vi "Table Info.vi"(8 "error in (no error)":errorcluster, 10 "table":string, 11 "SQLite3LV Cursor in":refnum<class "cursor.lvclass">) -> (0 "error out":errorcluster, 2 "table info.":T1[](array[typedef]), 3 "SQLite3LV Cursor out":refnum<class "cursor.lvclass">)   [LabVIEW 2014, in "SQLite3LV.lvlib" / "cursor.lvclass"]
doc: "A utility function that returns information about the specified table."
uses:
  cursor.lvclass
  SQLite3 Class/struct_table_info.ctl
  property binding/column I32.vi
  property binding/column Text.vi
  SQLite3LV.lvlib
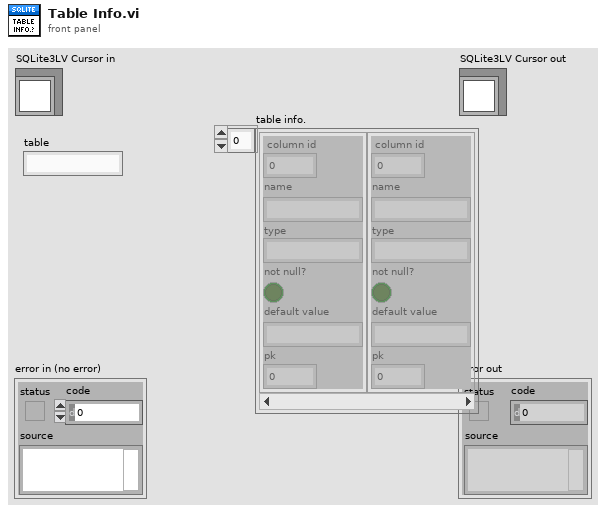
[diagram p1: front panel]
types:
  T1 = typedef "SQLite3LV.lvlib/struct_table_info.ctl" = cluster{" column id":i32, "name":string, "type":string, "not null?":bool, "default value":string, "pk":i32}
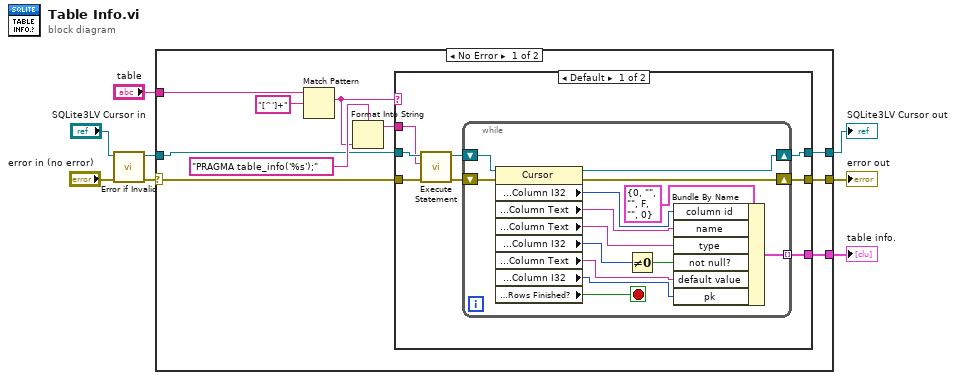
[diagram p0: block diagram]
diagram:
  n1 = call "Error if Invalid.vi"("error in (no error)"="error in (no error)", "SQLite3LV Cursor in"="SQLite3LV Cursor in") -> ("error out"=w1:errorcluster, "SQLite3LV Cursor out"=w2:refnum<class "cursor.lvclass">)  [unwired: 8 in]
  n2 = case shown="No Error" w1 {
    selector: w1 -> [w12 w44]
    tunnel: [w11 w44] -> w8
    tunnel: [w10 w43] -> w7
    tunnel: w2 -> [w13 w43]
    tunnel: "table" -> [w16 _]
    tunnel: [w9 _] -> w5
    frame No Error {
      n3 = Match Pattern(string=w16, regular expression="[^']+") -> (match substring=w15:string)  [unwired: 1 in, 3 out]
      n4 = Format Into String(format string="PRAGMA table_info('%s');", w15) -> (resulting string=w14:string)  [unwired: 2 in, 1 out]
      n5 = case shown="Default" w15 {
        tunnel: w14 -> [w25 _]
        tunnel: w13 -> [w26 w41]
        tunnel: w12 -> [w24 w42]
        tunnel: [w20 w42] -> w11
        tunnel: [w21 w41] -> w10
        tunnel: [w19 _] -> w9
        frame Default {
          n6 = call "Execute Statement.vi"("error in (no error)"=w24, "SQL statement"=w25, "SQLite3LV Cursor in"=w26) -> ("error out"=w22:errorcluster, "SQLite3LV Cursor out"=w23:refnum<class "cursor.lvclass">)  [unwired: 7 in]
          n7 = while {
            tunnel: [w32] -> w19 mode=indexing
            shift-right: [w29] -> w21
            shift-left: w23 -> [w40]
            shift-right: [w27] -> w20
            shift-left: w22 -> [w28]
            stop <- w31 stop-if-true
            n8 = property class="Cursor"(reference=w40, error in=w28) -> (reference out=w29:refnum<class "cursor.lvclass">, error out=w27:errorcluster, "property binding:Column I32"=w39:i32, "property binding:Column Text"=w35:string, "property binding:Column Text"=w36:string, "property binding:Column I32"=w38:i32, "property binding:Column Text"=w34:string, "property binding:Column I32"=w33:i32, "property binding:Rows Finished?"=w31:bool)
            n9 = Not Equal To 0?(x=w38) -> (x != 0?=w37:bool)
            n10 = Bundle By Name(cluster=T1 {" column id"=0, "name"="", "type"="", "not null?"=FALSE, "default value"="", "pk"=0} ("table info"), "column id"=w39, "name"=w35, "type"=w36, "not null?"=w37, "default value"=w34, "pk"=w33) -> (w32:T1)
          }
        }
        frame "" {
        }
      }
    }
    frame Error {
    }
  }
  "error out" <- w8
  "SQLite3LV Cursor out" <- w7
  "table info." <- w5
